vi "Draw Selection Prompt Text.vi"(7 "Bounds":T1={"left"=0, "top"=0, "right"=150, "bottom"=100}, 11 "Picture In":picture) -> (3 "Picture":picture)   [LabVIEW 2022 SP3, in "FlexBlocks Support.lvlib"]
uses:
  FlexBlocks Support.lvlib
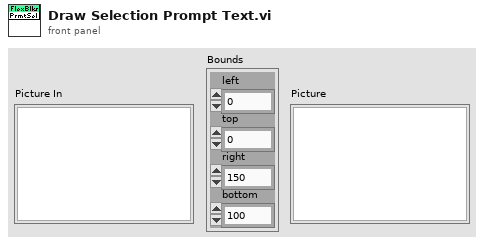
[diagram p1: front panel]
types:
  T1 = cluster{"left":i16, "top":i16, "right":i16, "bottom":i16}
  T2 = cluster{"horizontal":enum16{"left", "center", "right"}, "vertical":enum16{"top", "center", "bottom"}}
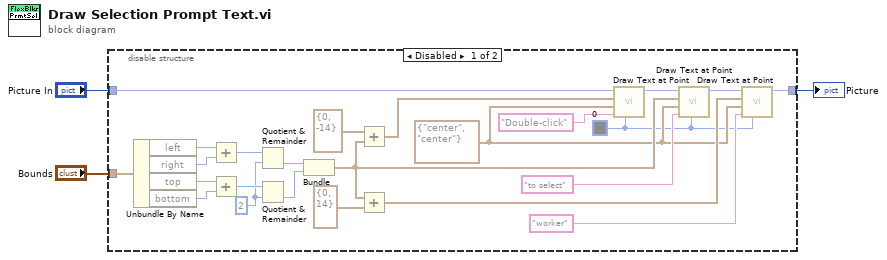
[diagram p0: block diagram]
diagram:
  n1 = disable-structure shown="Disabled" {
    disable-tunnel: "Picture In" -> [w27 w28]
    disable-tunnel: "Bounds" -> [w26 _]
    disable-tunnel: [w10 w28] -> w1
    frame Disabled {
      w4 = u32 0 ("text color(black)")
      w6 = T2 {"horizontal"=enum."center", "vertical"=enum."center"} ("alignment(left, top)")
      w19 = i16 2 ("y")
      n2 = Unbundle By Name(w26) -> ("left"=w25:i16, "right"=w24:i16, "top"=w23:i16, "bottom"=w22:i16)
      n3 = Add(x=w25, y=w24) -> (x+y=w21:i16)
      n4 = Add(x=w23, y=w22) -> (x+y=w20:i16)
      n5 = Quotient & Remainder(x=w21, y=w19) -> (floor(x/y)=w18:i16)  [unwired: 1 out]
      n6 = Quotient & Remainder(x=w20, y=w19) -> (floor(x/y)=w17:i16)  [unwired: 1 out]
      n7 = Bundle(w18, w17) -> (w8:cluster{i16, i16})  [unwired: 1 in]
      n8 = Add(x=cluster{i16, i16} {0, -14} ("output cluster"), y=w8) -> (x+y=w14:cluster{i16, i16})
      n9 = Add(x=w8, y=cluster{i16, i16} {0, 14} ("output cluster")) -> (x+y=w7:cluster{i16, i16})
      n10 = call <vilib>:"Draw Text at Point.vi"("text color(black)"=w4, "text"="Double-click", "alignment(left, top)"=w6, "origin"=w14, "picture"=w27) -> ("new picture"=w13:picture)  [unwired: 5 in, 1 out]
      n11 = call <vilib>:"Draw Text at Point.vi"("text color(black)"=w4, "text"="to select", "alignment(left, top)"=w6, "origin"=w8, "picture"=w13) -> ("new picture"=w11:picture)  [unwired: 5 in, 1 out]
      n12 = call <vilib>:"Draw Text at Point.vi"("text color(black)"=w4, "text"="worker", "alignment(left, top)"=w6, "origin"=w7, "picture"=w11) -> ("new picture"=w10:picture)  [unwired: 5 in, 1 out]
    }
    frame Enabled {
    }
  }
  "Picture" <- w1
